vi "PM-init.vi"(8 "error in (no error)":errorcluster) -> (0 "error out":errorcluster, 3 "init_cluster":T1)   [LabVIEW 2018]
uses:
  PM-init-data_cluster.ctl
  PM-init-user_events.ctl
  PM-common-heartrate_data.ctl
  PM-common-peak-detect_settings.ctl
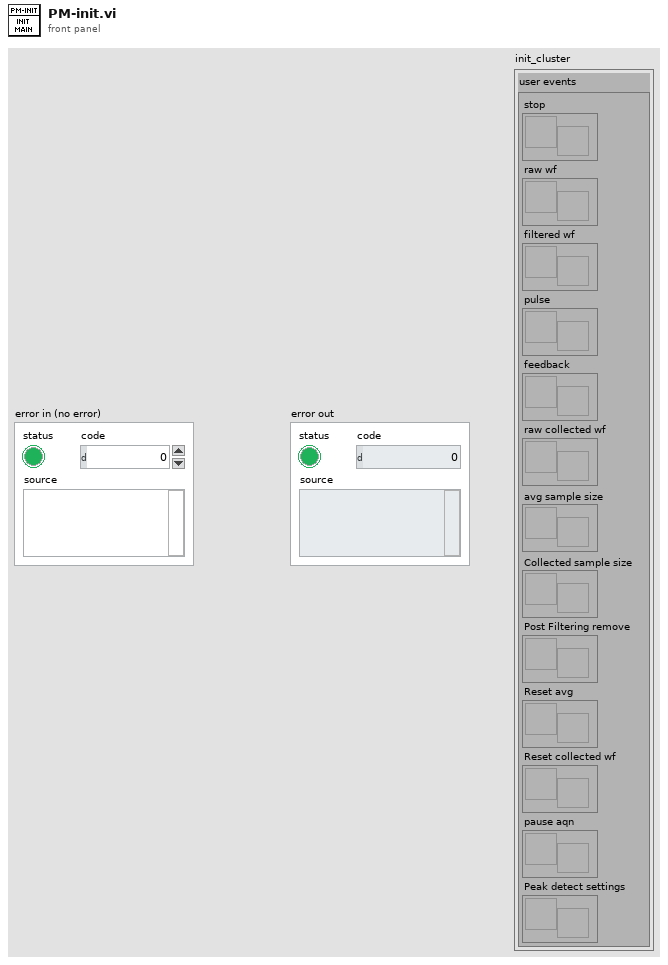
[diagram p1: front panel]
types:
  T1 = typedef "PM-init-data_cluster.ctl" = cluster{"user events":T2}
  T2 = typedef "PM-init-user_events.ctl" = cluster{"stop":refnum<user-event>, "raw wf":refnum<user-event>, "filtered wf":refnum<user-event>, "pulse":refnum<user-event>, "feedback":refnum<user-event>, "raw collected wf":refnum<user-event>, "avg sample size":refnum<user-event>, "Collected sample size":refnum<user-event>, "Post Filtering remove":refnum<user-event>, "Reset avg":refnum<user-event>, "Reset collected wf":refnum<user-event>, "pause aqn":refnum<user-event>, "Peak detect settings":refnum<user-event>}
  T3 = typedef "PM-common-peak-detect_settings.ctl" = cluster{"Top":dbl, "Bottom":dbl, "Peak Detection":bool}
  T4 = typedef "PM-common-heartrate_data.ctl" = cluster{"heartrate":dbl, "heartrate avg":dbl}
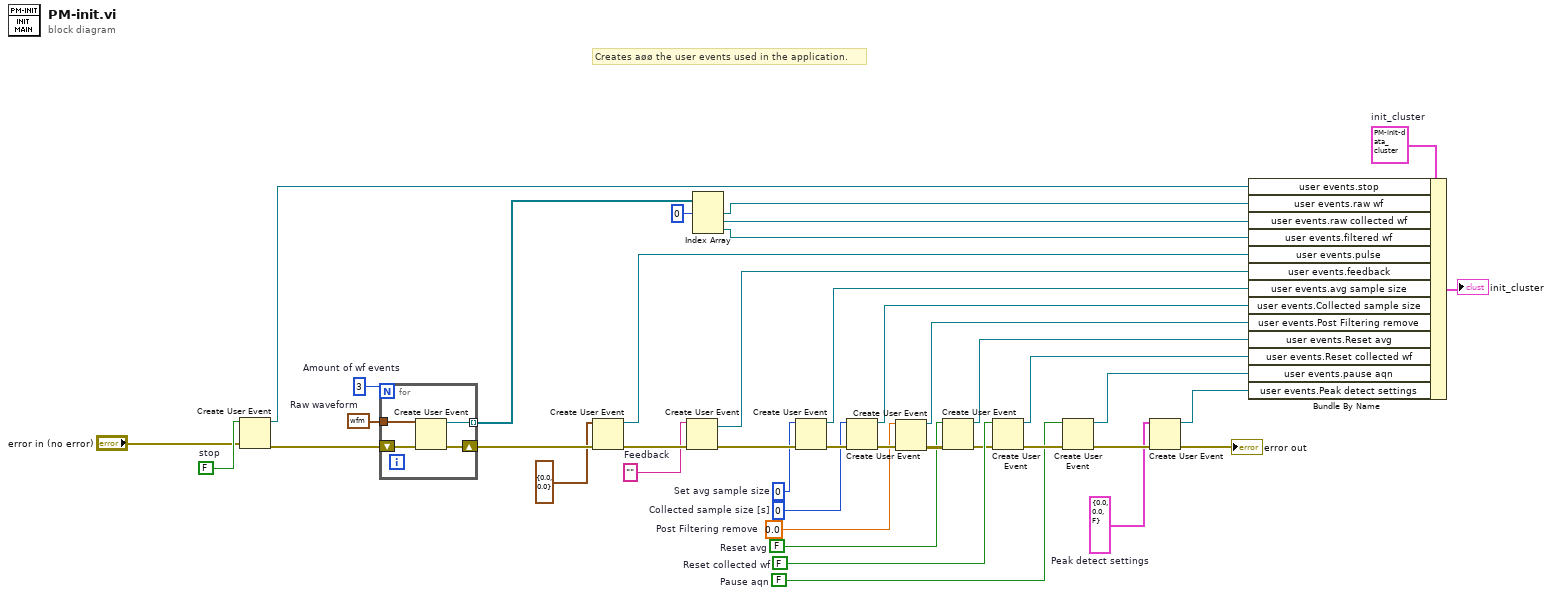
[diagram p0: block diagram]
diagram:
  w2 = T3 {"Top"=0.0, "Bottom"=0.0, "Peak Detection"=FALSE}  # Peak detect settings
  w6 = FALSE  # Pause aqn
  w14 = FALSE  # Reset collected wf
  w16 = 0.0  # Post Filtering remove
  w17 = u32 0  # Collected sample size [s]
  w15 = FALSE  # Reset avg
  w18 = u32 0  # Set avg sample size
  w25 = 3  # Amount of wf events
  w35 = ""  # Feedback
  w39 = FALSE  # stop
  w41 = T1 {"user events"={"stop"=refnum, "raw wf"=refnum, "filtered wf"=refnum, "pulse"=refnum, "feedback"=refnum, "raw collected wf"=refnum, "avg sample size"=refnum, "Collected sample size"=refnum, "Post Filtering remove"=refnum, "Reset avg"=refnum, "Reset collected wf"=refnum, "pause aqn"=refnum, "Peak detect settings"=refnum}}  # init_cluster
  w33 = waveform(dbl) {"t0"=timestamp(0 s since 1904-01-01), "dt"=1.0, "Y"=[]}  # Raw waveform
  # "Creates aøø the user events used in the application."
  n1 = Create User Event(user event datatype=w39, error in="error in (no error)") -> (user event=w38:refnum<user-event>, error out=w27:errorcluster)
  n2 = for {
    N: w25 -> [_]
    tunnel: w33 -> [w45]
    tunnel: [w44] -> w32 mode=indexing
    shift-right: [w43] -> w26
    shift-left: w27 -> [w42]
    n3 = Create User Event(user event datatype=w45, error in=w42) -> (user event=w44:refnum<user-event>, error out=w43:errorcluster)
  }
  n4 = Create User Event(user event datatype=T4 {"heartrate"=0.0, "heartrate avg"=0.0} ("heartrate data"), error in=w26) -> (user event=w23:refnum<user-event>, error out=w36:errorcluster)
  n5 = Create User Event(user event datatype=w35, error in=w36) -> (user event=w34:refnum<user-event>, error out=w22:errorcluster)
  n6 = Index Array(array=w32, index #1=0 ("index")) -> (element #1=w31:refnum<user-event>, element #2=w30:refnum<user-event>, element #3=w29:refnum<user-event>)  [unwired: 2 in]
  n7 = Create User Event(user event datatype=w18, error in=w22) -> (user event=w8:refnum<user-event>, error out=w21:errorcluster)
  n8 = Create User Event(user event datatype=w17, error in=w21) -> (user event=w12:refnum<user-event>, error out=w20:errorcluster)
  n9 = Create User Event(user event datatype=w16, error in=w20) -> (user event=w11:refnum<user-event>, error out=w19:errorcluster)
  n10 = Create User Event(user event datatype=w15, error in=w19) -> (user event=w10:refnum<user-event>, error out=w13:errorcluster)
  n11 = Create User Event(user event datatype=w14, error in=w13) -> (user event=w9:refnum<user-event>, error out=w7:errorcluster)
  n12 = Create User Event(user event datatype=w6, error in=w7) -> (user event=w5:refnum<user-event>, error out=w4:errorcluster)
  n13 = Create User Event(user event datatype=w2, error in=w4) -> (user event=w1:refnum<user-event>, error out=→"error out":errorcluster)
  n14 = Bundle By Name(cluster=w41, "user events.stop"=w38, "user events.raw wf"=w31, "user events.raw collected wf"=w30, "user events.filtered wf"=w29, "user events.pulse"=w23, "user events.feedback"=w34, "user events.avg sample size"=w8, "user events.Collected sample size"=w12, "user events.Post Filtering remove"=w11, "user events.Reset avg"=w10, "user events.Reset collected wf"=w9, "user events.pause aqn"=w5, "user events.Peak detect settings"=w1) -> (→"init_cluster":T1)
